vi "MoveToAxisTarget.vi"(8 "error in":errorcluster, 11 "axes":dbl[](array[numeric])) -> (0 "error out":errorcluster)   [LabVIEW 2013]
uses:
  CRCL Globals.vi
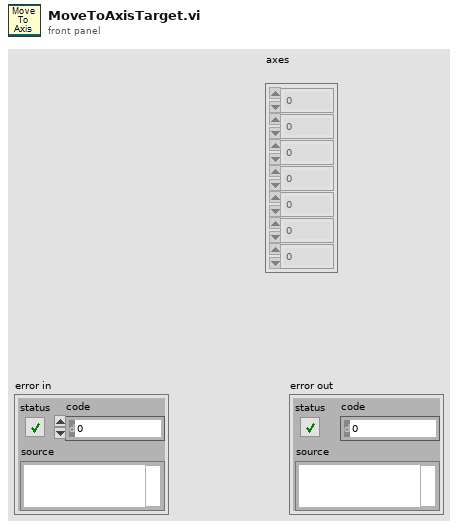
[diagram p1: front panel]
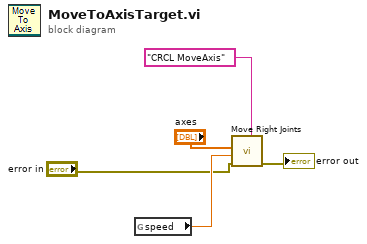
[diagram p0: block diagram]
diagram:
  n1 = global read "CRCL Globals.vi" "speed"() -> (w4:dbl)
  n2 = call "Move Right Joints.vi"("Label"="CRCL MoveAxis", "error in"="error in", "time"=w4, "Goal"="axes") -> ("error out"=→"error out":errorcluster)  [unwired: 7 in]
